vi "APLUS General Tester.vi"() -> ()   [LabVIEW 2016]
uses:
  <vilib>/NI/Modbus Library/API/Master/Modbus Master.lvclass
panel:
  in  "number of inputs":u16=2
  in  "starting address":u16
  out "word swapped":u32
  out "Numeric":sgl
  in  "Remote IP Address":string="192.168.1.101"
  in  "Remote Port":u16=502
  in  "error in (no error)":errorcluster
  in  "Reset WattHours":bool
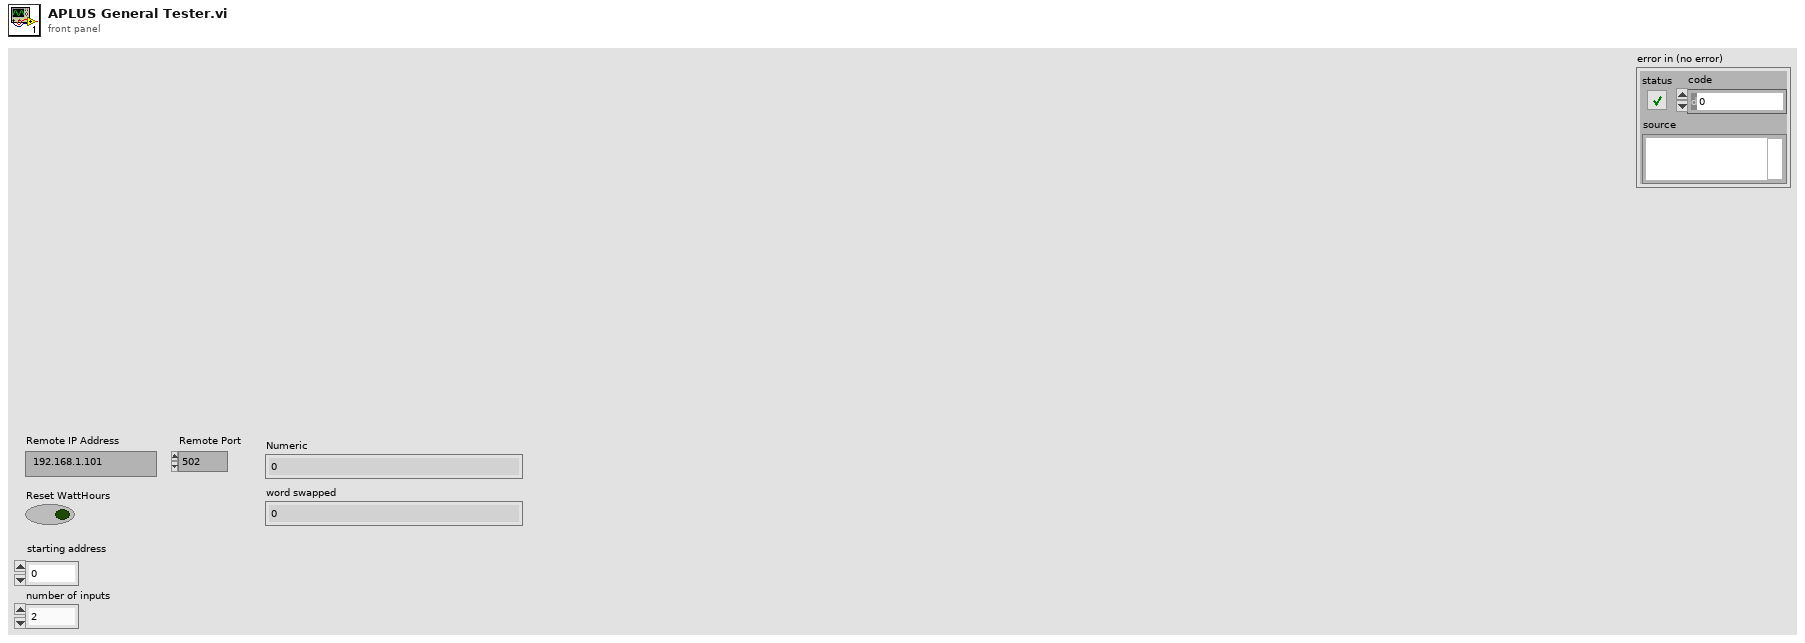
[diagram p1: front panel]
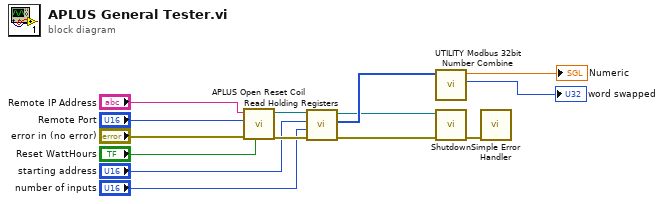
[diagram p0: block diagram]
diagram:
  n1 = call "APLUS Open Reset Coil.vi"("Reset WattHours"="Reset WattHours", "error in (no error)"="error in (no error)", "Remote Port"="Remote Port", "Remote IP Address"="Remote IP Address") -> ("error out"=w9:errorcluster, "Modbus Master out"=w8:refnum<class "Modbus Master.lvclass">)  [unwired: 6 in]
  n2 = call-dynamic "Read Holding Registers.vi"("error in"=w9, "number of inputs"="number of inputs", "starting address"="starting address", "Modbus master in"=w8) -> ("error out"=w7:errorcluster, "register values"=w10:u16[], "Modbus master out"=w6:refnum<class "Modbus Master.lvclass">)  [unwired: 5 in]
  n3 = call "UTILITY Modbus 32bit Number Combine.vi"("Holding Registers"=w10) -> ("word swapped"=→"word swapped":u32, "Data"=→"Numeric":sgl)  [unwired: 9 in]
  n4 = call-dynamic "Shutdown.vi"("error in"=w7, "Modbus master in"=w6) -> ("error out"=w5:errorcluster)  [unwired: 9 in]
  n5 = call <vilib>:"Simple Error Handler.vi"("error in (no error)"=w5) -> ()  [unwired: 1 in, 8 out]
